vi "New.vi"(8 "error in (no error)":errorcluster, 11 "PMU Configuration":T1) -> (0 "error out":errorcluster, 3 "Phasor Measurement Unit out":refnum<class "Phasor Measurement Unit.lvclass">)   [LabVIEW 2013, in "PMU Recorder Light.lvlib" / "Phasor Measurement Unit.lvclass"]
uses:
  Phasor Measurement Unit.lvclass
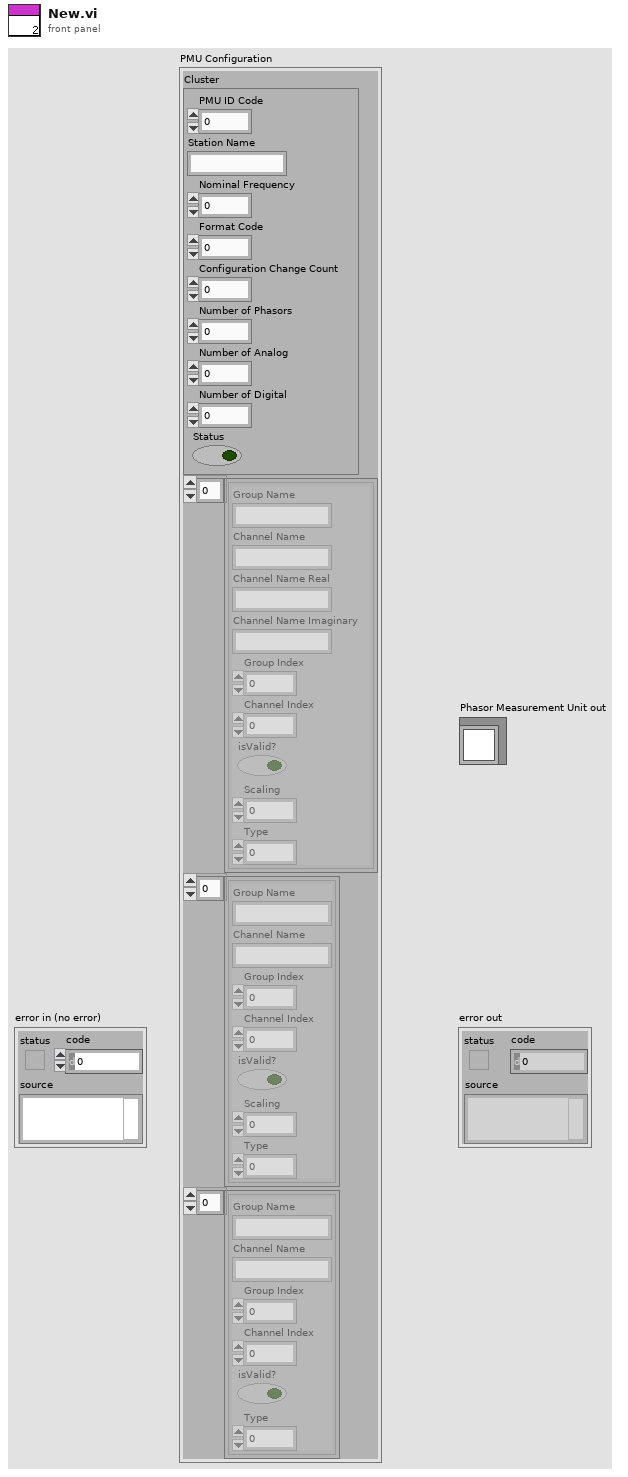
[diagram p1: front panel]
types:
  T1 = cluster{"Cluster":cluster{"PMU ID Code":i32, "Station Name":string, "Nominal Frequency":sgl, "Format Code":i32, "Configuration Change Count":i32, "Number of Phasors":i32, "Number of Analog":i32, "Number of Digital":i32, "Status":bool}, cluster{"Group Name":string, "Channel Name":string, "Channel Name Real":string, "Channel Name Imaginary":string, "Group Index":i32, "Channel Index":i32, "isValid?":bool, "Scaling":sgl, "Type":i32}[], cluster{"Group Name":string, "Channel Name":string, "Group Index":i32, "Channel Index":i32, "isValid?":bool, "Scaling":sgl, "Type":i32}[], cluster{"Group Name":string, "Channel Name":string, "Group Index":i32, "Channel Index":i32, "isValid?":bool, "Type":i32}[]}
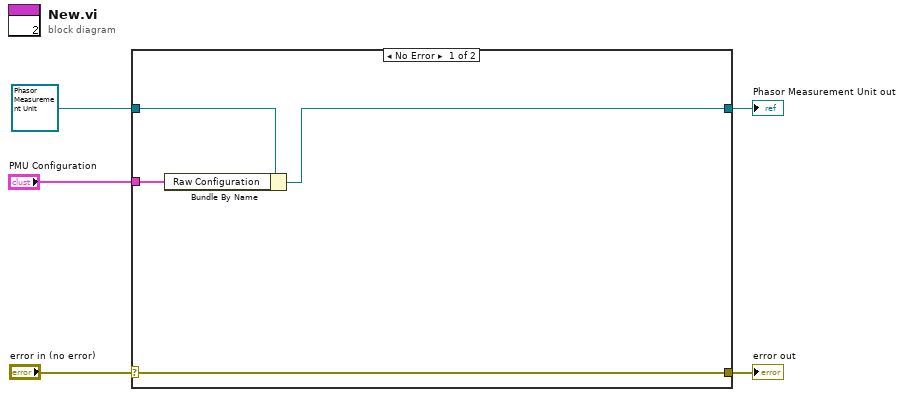
[diagram p0: block diagram]
diagram:
  n1 = case shown="No Error" "error in (no error)" {
    selector: "error in (no error)" -> [w9 w11]
    tunnel: [w9 w11] -> w4
    tunnel: [w6 w10] -> w3
    tunnel: refnum<class "Phasor Measurement Unit.lvclass"> refnum ("Phasor Measurement Unit in") -> [w7 w10]
    tunnel: "PMU Configuration" -> [w8 _]
    frame No Error {
      n2 = Bundle By Name(cluster=w7, "Raw Configuration"=w8) -> (w6:refnum<class "Phasor Measurement Unit.lvclass">)
    }
    frame Error {
    }
  }
  "error out" <- w4
  "Phasor Measurement Unit out" <- w3
